vi "TWM Wati for Measure End.vi"(0 "handle":i32, 1 "end of packet key":string="TWM:command:EndOfPacket", 3 "timeout [s] (10s)":dbl=30.0, 5 "meas root path (last)":path, 7 "quantity names (all)":string[](array[string]), 9 "stop ref (none)":refnum<vi>, 11 "error in":errorcluster, 12 "qwtb maxdim (scalar)":T3 caption="Max. shown dimension (scalar)", 13 "status ref (none)":refnum<vi>, 14 "phase ref channel tag (none)":string) -> (4 "handle out":i32, 6 "data":T2[][](array[typedef]), 8 "stoped?":bool, 10 "quantities":T1, 15 "error out":errorcluster)   [LabVIEW 2020]
doc: "TWM client top level function: Start measurement, wait for completion, Get result.\n\nSet reasonable timeout for the TWM sampling and processing. Wire in the the 'stop' reference to allow termination of the TWM task."
uses:
  external libraries/TWM client.lvlibp/server/TWM client/TWM Client Result Max Dim.ctl
  external libraries/TWM client.lvlibp/server/TWM client/TWM Client Quantity Record.ctl
  external libraries/TWM client.lvlibp/server/TWM client/TWM Client Result Info.ctl
  <vilib>/Utility/error.llb/Error Cluster From Error Code.vi
  <vilib>/ErrorRing/Error Ring.xnode
  external libraries/TWM client.lvlibp
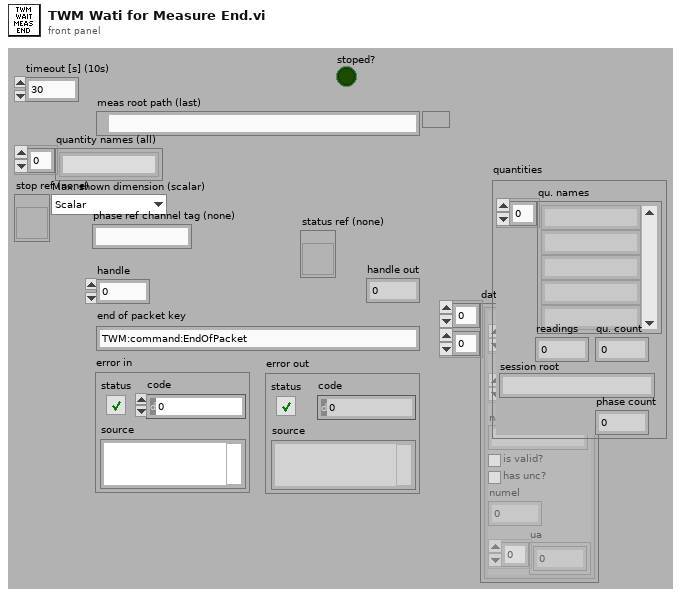
[diagram p1: front panel]
types:
  T1 = typedef "TWM client.lvlibp/TWM Client Result Info.ctl" = cluster{"qu. names":string[], "readings":i32, "qu. count":i32, "session root":string, "phase count":i32}
  T2 = typedef "TWM client.lvlibp/TWM Client Quantity Record.ctl" = cluster{"val":dbl[], "unc":dbl[], "name":string, "is valid?":bool, "has unc?":bool, "numel":i32, "ua":dbl[]}
  T3 = typedef "TWM client.lvlibp/TWM Client Result Max Dim.ctl" = enum16{"Scalar", "Vector", "Matrix"}
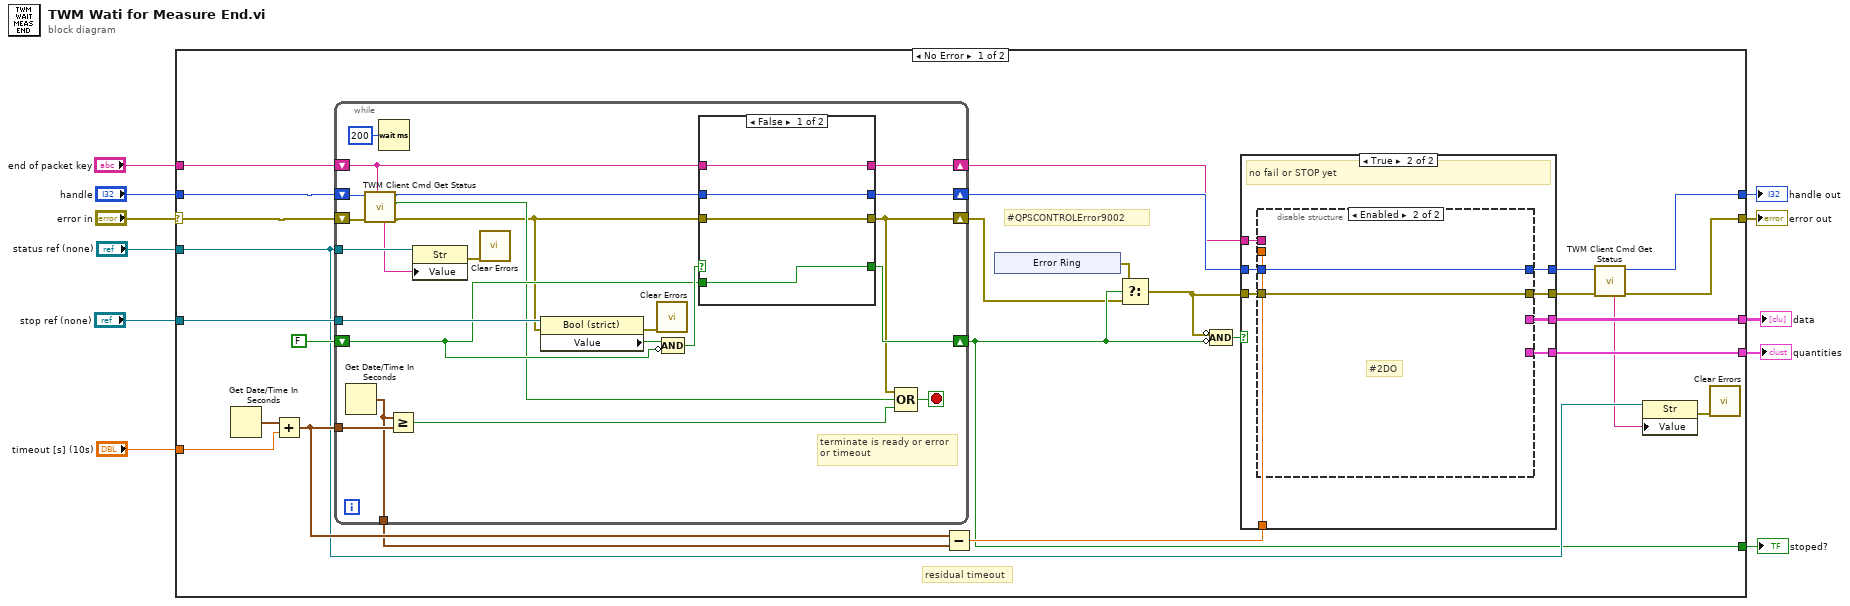
[diagram p0: block diagram]
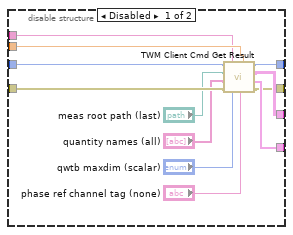
[diagram p3: hidden frame]
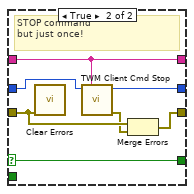
[diagram p4: hidden frame]
diagram:
  n1 = case shown="No Error" "error in" {
    selector: "error in" -> [w13 w102]
    tunnel: "handle" -> [w12 w101]
    tunnel: "stop ref (none)" -> [w37 _]
    tunnel: "timeout [s] (10s)" -> [w35 _]
    tunnel: "end of packet key" -> [w25 _]
    tunnel: [w23 w101] -> w7
    tunnel: [w21 w102] -> w6
    tunnel: [w27 _] -> w5
    tunnel: [w26 _] -> w4
    tunnel: [w17 _] -> w2
    tunnel: "status ref (none)" -> [w19 _]
    frame No Error {
      # "#QPSCONTROLError9002"
      # "residual timeout"
      n2 = Get Date/Time In Seconds() -> (seconds since 1Jan1904=w34:timestamp)
      n3 = Add(x=w34, y=w35) -> (x+y=w33:timestamp)
      n4 = while {
        shift-right: [w87] -> w30
        shift-left: w12 -> [w71]
        shift-right: [w81] -> w15
        shift-left: w13 -> [w72]
        tunnel: w37 -> [w88]
        shift-right: [w86] -> w17
        shift-left: FALSE -> [w83]
        tunnel: w33 -> [w82]
        tunnel: [w77] -> w32
        shift-right: [w76] -> w28
        shift-left: w25 -> [w70]
        tunnel: w19 -> [w69]
        stop <- w79 stop-if-true
        # "terminate is ready or error\nor timeout"
        n5 = Get Date/Time In Seconds() -> (seconds since 1Jan1904=w77:timestamp)
        n6 = call "TWM Client Cmd Get Status.vi"("end of packet key"=w70, "error in"=w72, "handle"=w71) -> ("error out"=w73:errorcluster, "ready?"=w74:bool, "handle out"=w75:i32, "status string"=w68:string)  [unwired: 4 in, 1 out]
        n7 = Wait (ms)(milliseconds to wait=u32 200) -> ()  [unwired: 1 out]
        n8 = Greater Or Equal?(x=w77, y=w82) -> (x >= y?=w80:bool)
        n9 = property class="Str"(reference=w69, "Value"=w68) -> (error out=w67:errorcluster)  [unwired: 1 in, 1 out]
        n10 = call <vilib>:"Clear Errors.vi"("error in (no error)"=w67) -> ()  [unwired: 5 in, 2 out]
        n11 = property class="Bool (strict)"(reference=w88, error in=w73) -> (error out=w89:errorcluster, "Value"=w85:bool)  [unwired: 1 out]
        n12 = call <vilib>:"Clear Errors.vi"("error in (no error)"=w89) -> ()  [unwired: 5 in, 2 out]
        n13 = Compound Arithmetic op=AND(w85, invert w83) -> (w84:bool)
        n14 = case shown="False" w84 {
          selector: w84 -> [_ w98]
          tunnel: w73 -> [w93 w100]
          tunnel: w75 -> [w92 w95]
          tunnel: [w92 w97] -> w87
          tunnel: [w93 w99] -> w81
          tunnel: [w91 w98] -> w86
          tunnel: w83 -> [w91 _]
          tunnel: w70 -> [w90 w96]
          tunnel: [w90 w96] -> w76
          frame False {
          }
          frame True {
            # "STOP command\nbut just once!"
            n15 = call <vilib>:"Clear Errors.vi"("error in (no error)"=w100) -> ()  [unwired: 5 in, 2 out]
            n16 = call "TWM Client Cmd Stop.vi"("end of packet key"=w96, "handle"=w95) -> ("error out"=w94:errorcluster, "handle out"=w97:i32)  [unwired: 8 in]
            n17 = Merge Errors(w100, w94) -> (w99:errorcluster)
          }
        }
        n18 = Compound Arithmetic op=OR(w81, w74, w80) -> (w79:bool)
      }
      n19 = Subtract(x=w33, y=w32) -> (x-y=w29:dbl)
      n20 = xnode "Error Ring"() -> ("error out"=w14:errorcluster)
      n21 = Select(t=w14, s=w17, f=w15) -> (s? t:f=w16:errorcluster)
      n22 = Compound Arithmetic op=AND(invert w16, invert w17) -> (w31:bool)
      n23 = case shown="True" w31 {
        tunnel: w16 -> [w44 w47]
        tunnel: w30 -> [w43 w52]
        tunnel: [w44 w48] -> w22
        tunnel: [w43 w51] -> w24
        tunnel: w29 -> [_ w46]
        tunnel: w28 -> [_ w45]
        tunnel: [_ w50] -> w27
        tunnel: [_ w49] -> w26
        frame False {
          # "STOP or error"
        }
        frame True {
          # "no fail or STOP yet"
          n24 = disable-structure shown="Enabled" {
            disable-tunnel: w52 -> [w64 w65]
            disable-tunnel: [w63 w65] -> w51
            disable-tunnel: [w62 _] -> w50
            disable-tunnel: [w61 _] -> w49
            disable-tunnel: [w60 w66] -> w48
            disable-tunnel: w47 -> [w59 w66]
            disable-tunnel: w46 -> [w54 _]
            disable-tunnel: w45 -> [w53 _]
            frame Disabled {
              n25 = call "TWM Client Cmd Get Result.vi"("phase ref channel tag (none)"="phase ref channel tag (none)", "timeout [s] (10s)"=w54, "qwtb maxdim (scalar)"="qwtb maxdim (scalar)", "end of packet key"=w53, "error in"=w59, "quantity names (all)"="quantity names (all)", "meas root path (last)"="meas root path (last)", "handle"=w64) -> ("error out"=w60:errorcluster, "result info"=w61:T1, "result data"=w62:T2[][], "handle out"=w63:i32)
            }
            frame Enabled {
              # "#2DO"
            }
          }
        }
      }
      n26 = call "TWM Client Cmd Get Status.vi"("error in"=w22, "handle"=w24) -> ("error out"=w21:errorcluster, "handle out"=w23:i32, "status string"=w18:string)  [unwired: 5 in, 2 out]
      n27 = property class="Str"(reference=w19, "Value"=w18) -> (error out=w20:errorcluster)  [unwired: 1 in, 1 out]
      n28 = call <vilib>:"Clear Errors.vi"("error in (no error)"=w20) -> ()  [unwired: 5 in, 2 out]
    }
    frame Error {
    }
  }
  "error out" <- w6
  "handle out" <- w7
  "data" <- w5
  "quantities" <- w4
  "stoped?" <- w2
